vi "Property Test.vi"   [LabVIEW 2016]
uses:
  Library/Classes/Manager/Memory.Manager.lvclass
  Library/Classes/Pointer/Memory.Pointer.lvclass
  Library/Classes/Pointer/Methods/Memory.Pointer.Allocate (32-bit).vi
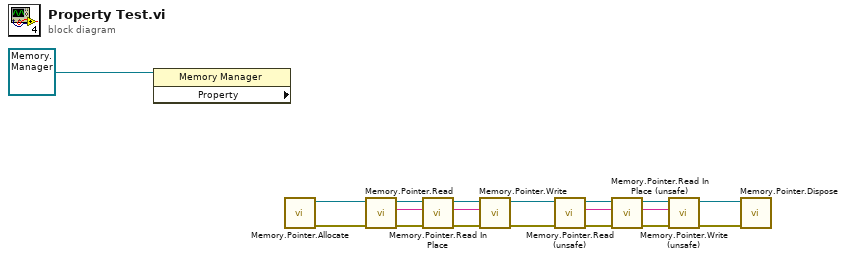
[diagram p0: block diagram]
diagram:
  n1 = property class="Memory Manager" props=[](reference=refnum<class "Memory.Manager.lvclass"> refnum ("LabVIEW Memory Manager.lvlib:Memory Manager")) -> ()  [unwired: 1 in, 3 out]
  n2 = call-poly "Memory.Pointer.Allocate.vi"() -> ("error out"=w17:errorcluster, "Pointer out"=w18:refnum<class "Memory.Pointer.lvclass">)  [unwired: 10 in]
  n3 = call "Memory.Pointer.Read.vi"("error in (no error)"=w17, "Pointer in"=w18) -> ("error out"=w15:errorcluster, "data"=w12:string, "Pointer out"=w16:refnum<class "Memory.Pointer.lvclass">)  [unwired: 7 in]
  n4 = call "Memory.Pointer.Read In Place.vi"("error in (no error)"=w15, "data in"=w12, "Pointer in"=w16) -> ("error out"=w13:errorcluster, "data out"=w11:string, "Pointer out"=w14:refnum<class "Memory.Pointer.lvclass">)  [unwired: 6 in]
  n5 = call "Memory.Pointer.Write.vi"("error in (no error)"=w13, "data"=w11, "Pointer in"=w14) -> ("error out"=w9:errorcluster, "Pointer out"=w10:refnum<class "Memory.Pointer.lvclass">)  [unwired: 6 in, 1 out]
  n6 = call "Memory.Pointer.Read (unsafe).vi"("error in (no error)"=w9, "Pointer in"=w10) -> ("error out"=w7:errorcluster, "data"=w3:string, "Pointer out"=w8:refnum<class "Memory.Pointer.lvclass">)  [unwired: 7 in]
  n7 = call "Memory.Pointer.Read In Place (unsafe).vi"("error in (no error)"=w7, "data in"=w3, "Pointer in"=w8) -> ("error out"=w5:errorcluster, "data out"=w1:string, "Pointer out"=w6:refnum<class "Memory.Pointer.lvclass">)  [unwired: 6 in]
  n8 = call "Memory.Pointer.Write (unsafe).vi"("error in (no error)"=w5, "data"=w1, "Pointer in"=w6) -> ("error out"=w4:errorcluster, "Pointer out"=w2:refnum<class "Memory.Pointer.lvclass">)  [unwired: 6 in, 1 out]
  n9 = call "Memory.Pointer.Dispose.vi"("error in (no error)"=w4, "Pointer in"=w2) -> ()  [unwired: 9 in, 1 out]
